vi "SetPIDAngleGains.vi"(10 "Angle PID gains":T1, 11 "DriveBase.lvclass":refnum<class "DriveBase.lvclass">) -> (3 "DriveBase.lvclass 2":refnum<class "DriveBase.lvclass">)   [LabVIEW 2016, in "DriveBase.lvclass"]
uses:
  DriveBase.lvclass
  DriveBase.lvclass/DriveBase.ctl
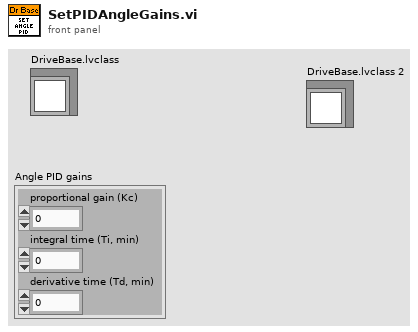
[diagram p1: front panel]
types:
  T1 = cluster{"proportional gain (Kc)":dbl, "integral time (Ti, min)":dbl, "derivative time (Td, min)":dbl}
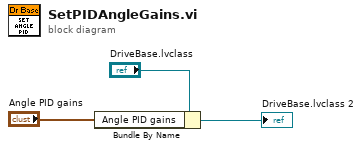
[diagram p0: block diagram]
diagram:
  n1 = Bundle By Name(cluster="DriveBase.lvclass", "Angle PID gains"="Angle PID gains") -> (→"DriveBase.lvclass 2":refnum<class "DriveBase.lvclass">)
